vi "joystick deadzone.vi"(8 "minpower":dbl, 9 "deadzone":dbl, 11 "joystick":dbl) -> (3 "joyout":dbl)   [LabVIEW 2014]
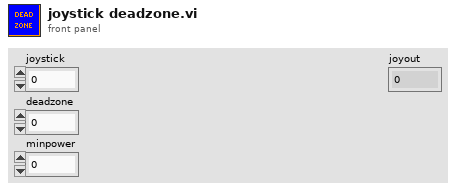
[diagram p1: front panel]
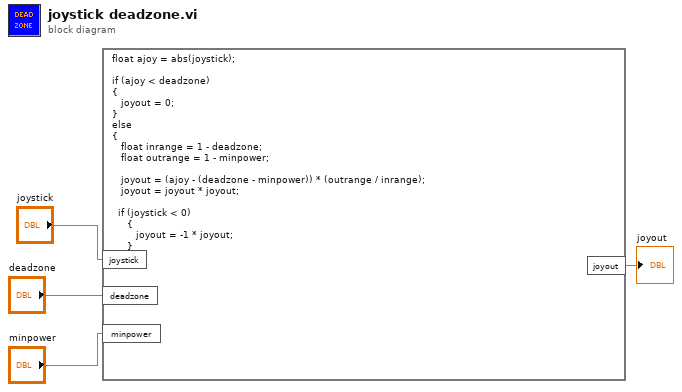
[diagram p0: block diagram]
diagram:
  n1 = formula code="float ajoy = abs(joystick);\n\nif (ajoy < deadzone)\n{\n   joyout = 0;\n}\nelse\n{\n   float inrange = 1 - deadzone;\n   float outrange = 1 - minpower;\n\n   joyout = (ajoy - (deadzone - minpower)) * (outrange / inrange);\n   joyout = joyout * joyout;\n\n  if (joystick < 0)\n     {\n        joyout = -1 * joyout;\n     }\n}"("joystick"="joystick", "deadzone"="deadzone", "minpower"="minpower") -> ("joyout"=→"joyout":dbl)
